vi "thruster_thrust_dir_set.vi"(7 "index":u16, 8 "Forward":bool, 9 "Thrust":u16, 10 "Address":u16, 11 "VISA resource name":refnum<visa-resource-name>) -> ()   [LabVIEW 2014]
panel:
  in  "Addres":u16
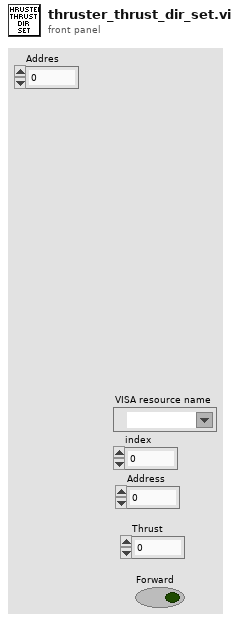
[diagram p1: front panel]
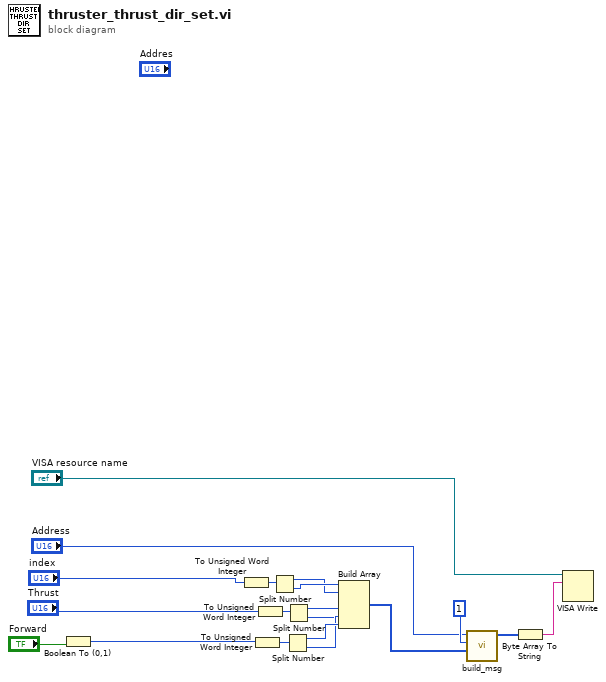
[diagram p0: block diagram]
diagram:
  n1 = Boolean To (0,1)(Boolean="Forward") -> (0, 1=w7:i16)
  n2 = To Unsigned Word Integer(number="index") -> (unsigned 16bit integer=w4:u16)
  n3 = To Unsigned Word Integer(number=w7) -> (unsigned 16bit integer=w13:u16)
  n4 = To Unsigned Word Integer(number="Thrust") -> (unsigned 16bit integer=w19:u16)
  n5 = Split Number(x=w4) -> (hi(x)=w2:u8, lo(x)=w3:u8)
  n6 = Split Number(x=w13) -> (hi(x)=w17:u8, lo(x)=w16:u8)
  n7 = Split Number(x=w19) -> (hi(x)=w15:u8, lo(x)=w14:u8)
  n8 = Build Array(w3, w2, w14, w15, w16, w17) -> (w18:u8[])
  n9 = call "build_msg.vi"("data"=w18, "ID"=u16 1, "Address"="Address") -> ("msg"=w11:u8[])  [unwired: 8 in]
  n10 = Byte Array To String(unsigned byte array=w11) -> (string=w10:string)
  n11 = VISA Write(VISA resource name="VISA resource name", write buffer=w10) -> ()  [unwired: 1 in, 3 out]
